vi "IMAQ-U32RGB.vi"(0 "Image Pixels (RGB32) 2D Array":u32[][](array[numeric])) -> (1 "Blue 2D Array":dbl[][](array[numeric]), 2 "Green 2D Array":dbl[][](array[numeric]), 3 "Red 2D Array":dbl[][](array[numeric]))   [LabVIEW 2010]
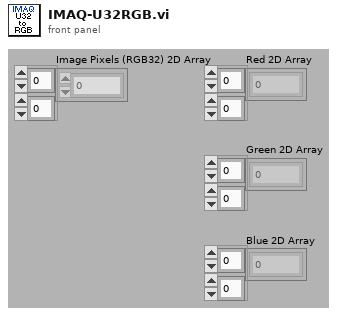
[diagram p1: front panel]
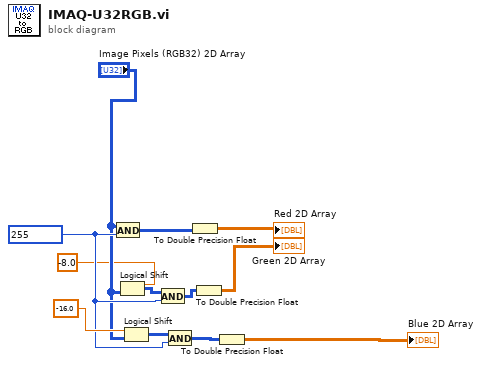
[diagram p0: block diagram]
diagram:
  w6 = u32 255
  n1 = And(x="Image Pixels (RGB32) 2D Array", y=w6) -> (x .and. y?=w1:u32[][])
  n2 = Logical Shift(y=sgl -8.0 ("x"), x="Image Pixels (RGB32) 2D Array") -> (x << y=w4:u32[][])
  n3 = Logical Shift(y=sgl -16.0 ("x"), x="Image Pixels (RGB32) 2D Array") -> (x << y=w5:u32[][])
  n4 = And(x=w4, y=w6) -> (x .and. y?=w7:u32[][])
  n5 = And(x=w5, y=w6) -> (x .and. y?=w8:u32[][])
  n6 = To Double Precision Float(number=w1) -> (double precision float=→"Red 2D Array":dbl[][])
  n7 = To Double Precision Float(number=w7) -> (double precision float=→"Green 2D Array":dbl[][])
  n8 = To Double Precision Float(number=w8) -> (double precision float=→"Blue 2D Array":dbl[][])
